vi "Ticks delay to trig delay.vi"() -> ()   [LabVIEW 2019]
panel:
  out "actual delay":dbl
  out "ticks":dbl
  in  "dt":dbl format="%#_6p"
  in  "delay":dbl format="%#_6p"
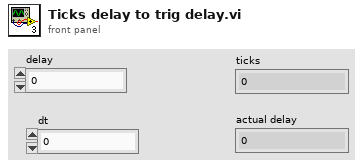
[diagram p1: front panel]
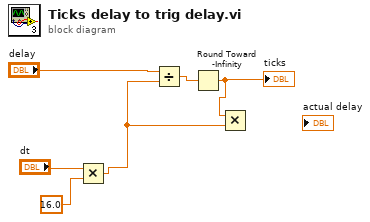
[diagram p0: block diagram]
diagram:
  n1 = Multiply(x="dt", y=16.0) -> (x*y=w1:dbl)
  n2 = Divide(x="delay", y=w1) -> (x/y=w3:dbl)
  n3 = Round Toward -Infinity(1:w3) -> (0:w2:dbl)
  "ticks" <- w2
  n4 = Multiply(x=w2, y=w1) -> ()  [unwired: 1 out]
